vi "Arm.vi"() -> ()   [LabVIEW 2017]
uses:
  <vilib>/Rock Robotics/WPI/ThirdParty/Phoenix-LabVIEW/Motor Controller/Controls/CTRE_Phoenix_MotorControl_ControlMode.ctl
  <vilib>/Rock Robotics/WPI/Utilities/WPI_GetSetVariantRefNum.vi
  Robot Global Data.vi
  <vilib>/Rock Robotics/WPI/ThirdParty/Phoenix-LabVIEW/Motor Controller/Get/CTRE_Phoenix_MotorController_GetPulseWidthAll.vi
panel:
  out "Position (Degrees)":i32
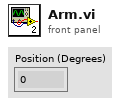
[diagram p1: front panel]
types:
  T1 = typedef "WPI_MotorControlDeviceRef.ctl" = cluster{"DeviceStatus":errorcluster, "Type":T2, "PWM":cluster{"PWM Channel":T3, "DeadBand":T4}, "CAN":cluster{"Device Number":u8, "SetOutput VI Ref":variant, "GetOutput VI Ref":variant, "Enable VI Ref":variant, "Disable VI Ref":variant, "Data":variant}, "Invert":bool, "DIO PWM":cluster{"PWM \"Enable\" Channel":T3, "DIOChannel":T5, "PWM Rate":dbl}}
  T2 = typedef "WPI_MotorControlType.ctl" = enum16{"PWM", "CAN", "DIO PWM"}
  T3 = typedef "FPGA_DIOPWMChannel.ctl" = enum8{"PWM 0", "PWM 1", "PWM 2", "PWM 3", "PWM 4", "PWM 5", "PWM 6", "PWM 7", "PWM 8", "PWM 9", "PWM MXP 0", "PWM MXP 1", "PWM MXP 2", "PWM MXP 3", "PWM MXP 4", "PWM MXP 5", "PWM MXP 6", "PWM MXP 7", "PWM MXP 8", "PWM MXP 9", "Invalid"}
  T4 = typedef "WPI_PWMDeadband.ctl" = cluster{"Name":string, "maxPositivePwm":i32, "minPositivePwm":i32, "centerPwm":i32, "maxNegativePwm":i32, "minNegativePwm":i32, "angularRange":u16}
  T5 = typedef "FPGA_DIOChannel.ctl" = enum8{"DIO 0", "DIO 1", "DIO 2", "DIO 3", "DIO 4", "DIO 5", "DIO 6", "DIO 7", "DIO 8", "DIO 9", "DIO MXP 0", "DIO MXP 1", "DIO MXP 2", "DIO MXP 3", "DIO MXP 4", "DIO MXP 5", "DIO MXP 6", "DIO MXP 7", "DIO MXP 8", "DIO MXP 9", "DIO MXP 10", "DIO MXP 11", "DIO MXP 12", "DIO MXP 13", "DIO MXP 14", "DIO MXP 15", "SPI Port CS1", "SPI Port CS2", "SPI Port CS3", "SPI Port MISO", "SPI Port MOSI", "Invalid"}
  T6 = typedef "WPI_JoystickDevRef.ctl" = cluster{"Device":T7}
  T7 = typedef "WPI_JoystickDeviceEnum.ctl" = enum16{"USB 0", "USB 1", "USB 2", "USB 3", "USB 4", "USB 5"}
  T8 = typedef "CTRE_Phoenix_MotorControl_ControlMode.ctl" = u16
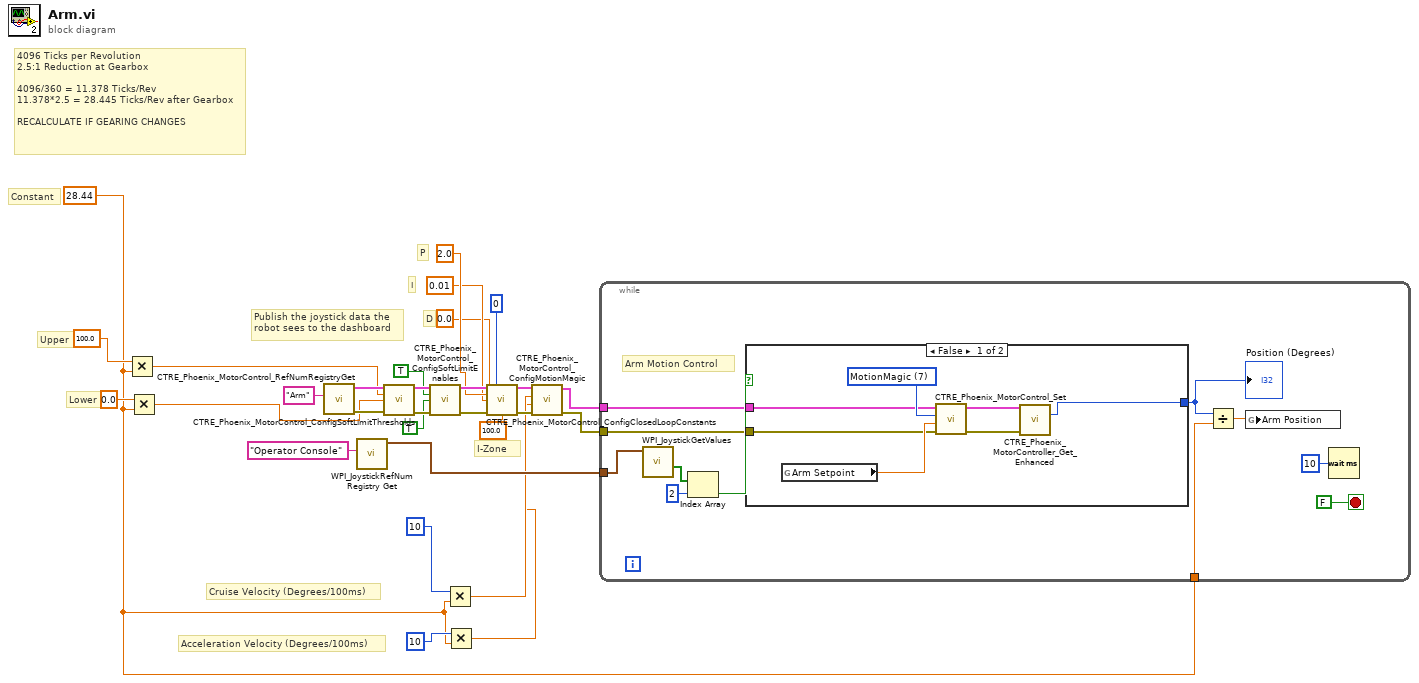
[diagram p0: block diagram]
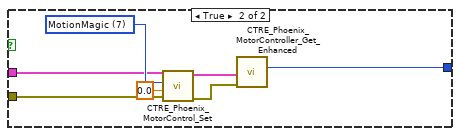
[diagram p2: hidden frame]
diagram:
  w2 = 28.44 ("y")
  # "I-Zone"
  # "D"
  # "I"
  # "P"
  # "Acceleration Velocity (Degrees/100ms)"
  # "Cruise Velocity (Degrees/100ms)"
  # "Lower"
  # "Upper"
  # "Constant"
  # "4096 Ticks per Revolution\n2.5:1 Reduction at Gearbox\n\n4096/360 = 11.378 Ticks/Rev\n11.378*2.5 = 28.445 Ticks/Rev after Gearbox\n\nRECALCULATE IF GEARING CHANGES"
  # "Publish the joystick data the\nrobot sees to the dashboard"
  n1 = Multiply(x=100.0, y=w2) -> (x*y=w8:dbl)
  n2 = Multiply(x=0.0, y=w2) -> (x*y=w7:dbl)
  n3 = call <vilib>:"CTRE_Phoenix_MotorControl_RefNumRegistryGet.vi"("refnum name"="Arm") -> ("error out"=w26:errorcluster, "PhoenixMotorControlDevRef"=w27:T1)  [unwired: 9 in]
  n4 = call <vilib>:"WPI_JoystickRefNum Registry Get.vi"("refnum name"="Operator Console") -> ("JoystickDevRef"=w15:T6)  [unwired: 1 in, 9 out]
  n5 = call <vilib>:"CTRE_Phoenix_MotorControl_ConfigSoftLimitThresholds.vi"("PhoenixMotorControlDevRef"=w27, "Forward Soft Limit"=w8, "Reverse Soft Limit"=w7, "error in (no error)"=w26) -> ("PhoenixMotorControlDevRef"=w25:T1, "error out"=w24:errorcluster)  [unwired: 10 in]
  n6 = call <vilib>:"CTRE_Phoenix_MotorControl_ConfigSoftLimitEnables.vi"("PhoenixMotorControlDevRef"=w25, "Forward Soft Limit Enable"=TRUE, "Reverse Soft Limit Enable"=TRUE, "error in (no error)"=w24) -> ("PhoenixMotorControlDevRef"=w21:T1, "error out"=w20:errorcluster)  [unwired: 10 in]
  n7 = Multiply(x=10 ("Cruise Velocity"), y=w2) -> (x*y=w4:dbl)
  n8 = Multiply(x=10 ("Acceleration"), y=w2) -> (x*y=w3:dbl)
  n9 = call <vilib>:"CTRE_Phoenix_MotorControl_ConfigClosedLoopConstants.vi"("PhoenixMotorControlDevRef"=w21, "slotIdx"=0, "P"=2.0, "I"=0.01, "D"=0.0, "error in (no error)"=w20, "I Zone"=100.0) -> ("PhoenixMotorControlDevRef"=w14:T1, "error out"=w13:errorcluster)  [unwired: 7 in]
  n10 = call <vilib>:"CTRE_Phoenix_MotorControl_ConfigMotionMagic.vi"("error in (no error)"=w13, "Acceleration"=w3, "Cruise Velocity"=w4, "PhoenixMotorControlDevRef"=w14) -> ("error out"=w11:errorcluster, "PhoenixMotorControlDevRef"=w12:T1)  [unwired: 6 in]
  n11 = while {
    tunnel: w15 -> [w38]
    tunnel: w12 -> [w34]
    tunnel: w11 -> [w33]
    tunnel: w2 -> [w30]
    stop <- FALSE stop-if-true
    # "Arm Motion Control"
    n12 = call <vilib>:"WPI_JoystickGetValues.vi"("JoystickDevRef"=w38) -> ("Buttons"=w37:bool[])  [unwired: 6 in, 4 out]
    n13 = Index Array(array=w37, index=2) -> (element=w35:bool)
    n14 = case shown="False" w35 {
      tunnel: [w44 w51] -> w32
      tunnel: w34 -> [w42 w50]
      tunnel: w33 -> [w41 w49]
      frame False {
        w47 = T8 7 items=["PercentOutput"=0, "Position"=1, "Velocity"=2, "Current"=3, "Follower"=5, "MotionProfile"=6, "MotionMagic"=7, "MotionMagicArc"=8, "MotionProfileArc"=10, "Disabled"=15] ("Control Mode")
        n15 = global read "Robot Global Data.vi" "Arm Setpoint"() -> (w43:dbl)
        n16 = call <vilib>:"CTRE_Phoenix_MotorControl_Set.vi"("error in (no error)"=w41, "Output"=w43, "Control Mode"=w47, "PhoenixMotorControlDevRef"=w42) -> ("error out"=w45:errorcluster, "PhoenixMotorControlDevRef"=w46:T1)  [unwired: 6 in]
        n17 = call-poly <vilib>:"CTRE_Phoenix_MotorController_Get_Enhanced.vi"("PhoenixMotorControlDevRef"=w46, "error in"=w45) -> ("Pulse Width Position"=w44:i32)  [unwired: 8 in, 5 out]
      }
      frame True {
        w54 = T8 7 items=["PercentOutput"=0, "Position"=1, "Velocity"=2, "Current"=3, "Follower"=5, "MotionProfile"=6, "MotionMagic"=7, "MotionMagicArc"=8, "MotionProfileArc"=10, "Disabled"=15] ("Control Mode")
        n18 = call <vilib>:"CTRE_Phoenix_MotorControl_Set.vi"("error in (no error)"=w49, "Output"=0.0, "Control Mode"=w54, "PhoenixMotorControlDevRef"=w50) -> ("error out"=w52:errorcluster, "PhoenixMotorControlDevRef"=w53:T1)  [unwired: 6 in]
        n19 = call-poly <vilib>:"CTRE_Phoenix_MotorController_Get_Enhanced.vi"("PhoenixMotorControlDevRef"=w53, "error in"=w52) -> ("Pulse Width Position"=w51:i32)  [unwired: 8 in, 5 out]
      }
    }
    "Position (Degrees)" <- w32
    n20 = Divide(x=w32, y=w30) -> (x/y=w31:dbl)
    n21 = global write "Robot Global Data.vi" "Arm Position"(w31) -> ()
    n22 = Wait (ms)(milliseconds to wait=u32 10) -> ()  [unwired: 1 out]
  }
